vi "Collect Blueprints.vi"(1 "Blueprints List":string="Blueprint 1: Each ore robot costs 4 ore. Each clay robot costs 2 ore. Each obsidian robot costs 3 ore and 14 clay. Each geode robot costs 2 ore and 7 obsidian.\nBlueprint 2: Each ore robot costs 2 ore. Each clay robot costs 3 ore. Each obsidian robot costs 3 ore and 8 clay. Each geode robot costs 3 ore and 12 obsidian.") -> (0 "Blueprints":T1 {"Robot Building Costs"."Geode"."Mineral" items=["Ore", "Clay", "Obsidian", "Geode", "Open Geode"]; "Robot Building Costs"."Obsidian"."Mineral" items=["Ore", "Clay", "Obsidian", "Geode", "Open Geode"]; "Robot Building Costs"."Clay"."Mineral" items=["Ore", "Clay", "Obsidian", "Geode", "Open Geode"]; "Robot Building Costs"."Ore"."Mineral" items=["Ore", "Clay", "Obsidian", "Geode", "Open Geode"]})   [LabVIEW 2020, in "AoC 2022.lvlib"]
uses:
  AoC 2022.lvlib
  Blueprints.ctl
  Robot Building Costs.ctl
  Cost.ctl
  Mineral.ctl
  Mineral_Enum.ctl
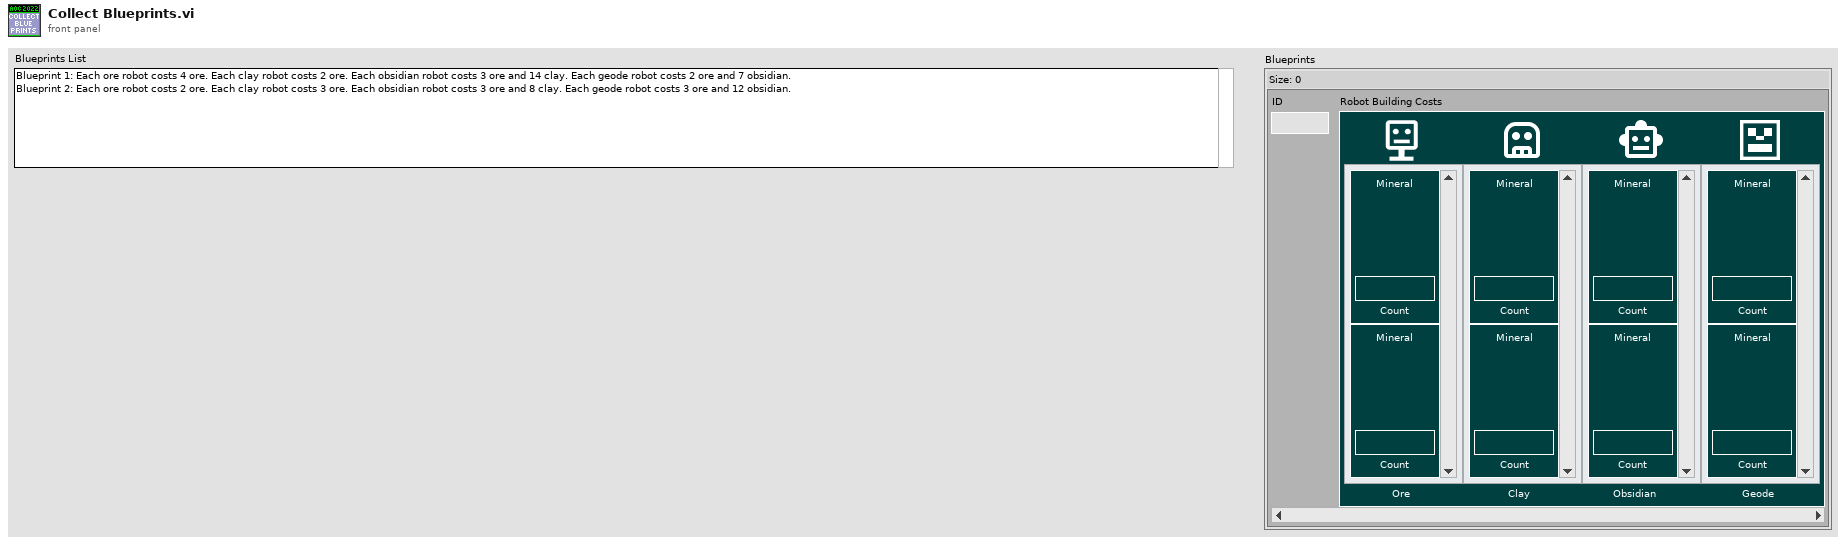
[diagram p1: front panel]
types:
  T1 = typedef "AoC 2022.lvlib/Blueprints.ctl" = map{i32, T2}
  T2 = typedef "AoC 2022.lvlib/Robot Building Costs.ctl" = cluster{"Ore":T3[], "Clay":T3[], "Obsidian":T3[], "Geode":T3[]}
  T3 = typedef "AoC 2022.lvlib/Cost.ctl" = cluster{"Mineral":T4, "Count":u32}
  T4 = typedef "AoC 2022.lvlib/Mineral.ctl" = u16
  T5 = typedef "AoC 2022.lvlib/Mineral_Enum.ctl" = enum16{"ore", "clay", "obsidian", "geode", "Open Geode"}
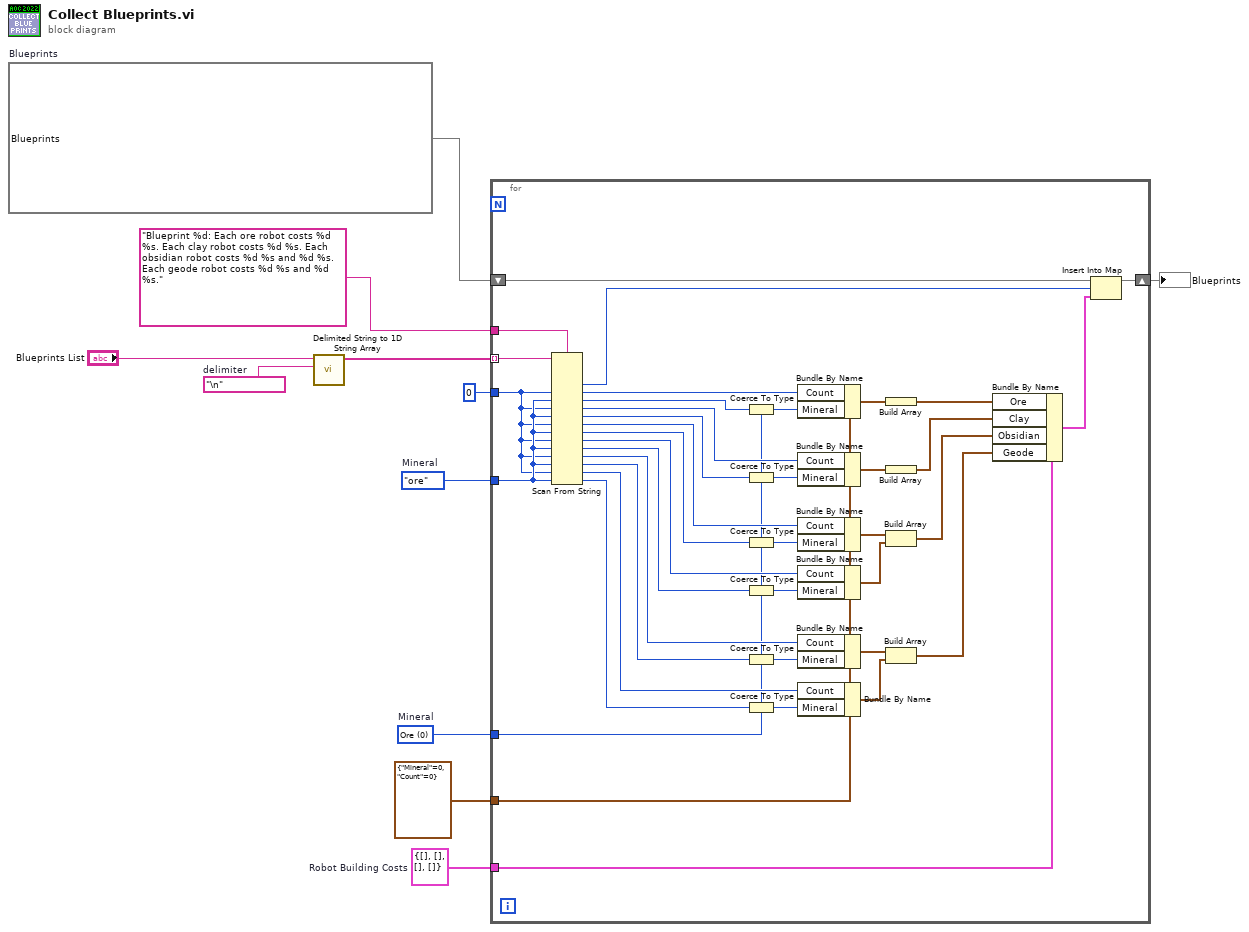
[diagram p0: block diagram]
diagram:
  w2 = T4 0 items=["Ore", "Clay", "Obsidian", "Geode", "Open Geode"]  # Mineral
  w4 = T2 {"Ore"=[], "Clay"=[], "Obsidian"=[], "Geode"=[]}  # Robot Building Costs
  w6 = T1 {}  # Blueprints
  w7 = Mineral_Enum."ore"  # Mineral
  w10 = "\n"  # delimiter
  n1 = call <vilib>:"Delimited String to 1D String Array.vi"("delimiter"=w10, "delimited string"="Blueprints List") -> ("string array"=w11:string[])  [unwired: 9 in]
  n2 = for {
    tunnel: w11 -> [w50] mode=indexing
    tunnel: "Blueprint %d: Each ore robot costs %d %s. Each clay robot costs %d %s. Each obsidian robot costs %d %s and %d %s. Each geode robot costs %d %s and %d %s." -> [w49]
    tunnel: w7 -> [w43]
    shift-right: [w47] -> w1
    shift-left: w6 -> [w48]
    tunnel: u32 0 -> [w22]
    tunnel: w4 -> [w45]
    tunnel: T3 {"Mineral"=0, "Count"=0} ("Cost") -> [w40]
    tunnel: w2 -> [w23]
    n3 = Scan From String(format string=w49, input string=w50, default 2=w22, default 3=w43, default 4=w22, default 5=w43, default 6=w22, default 7=w43, default 8=w22, default 9=w43, default 10=w22, default 11=w43, default 12=w22, default 13=w43) -> (output 1=w46:i32, output 2=w42:u32, output 3=w41:T5, output 4=w39:u32, output 5=w38:T5, output 6=w37:u32, output 7=w36:T5, output 8=w35:u32, output 9=w34:T5, output 10=w33:u32, output 11=w32:T5, output 12=w31:u32, output 13=w30:T5)  [unwired: 3 in, 3 out]
    n4 = Coerce To Type(0:w41, 1:w23) -> (2:w28:T4)
    n5 = Coerce To Type(0:w38, 1:w23) -> (2:w29:T4)
    n6 = Coerce To Type(0:w36, 1:w23) -> (2:w27:T4)
    n7 = Coerce To Type(0:w34, 1:w23) -> (2:w26:T4)
    n8 = Coerce To Type(0:w32, 1:w23) -> (2:w25:T4)
    n9 = Coerce To Type(0:w30, 1:w23) -> (2:w24:T4)
    n10 = Bundle By Name(cluster=w40, "Count"=w42, "Mineral"=w28) -> (w21:T3)
    n11 = Bundle By Name(cluster=w40, "Count"=w39, "Mineral"=w29) -> (w19:T3)
    n12 = Bundle By Name(cluster=w40, "Count"=w37, "Mineral"=w27) -> (w18:T3)
    n13 = Bundle By Name(cluster=w40, "Count"=w35, "Mineral"=w26) -> (w15:T3)
    n14 = Bundle By Name(cluster=w40, "Count"=w33, "Mineral"=w25) -> (w14:T3)
    n15 = Bundle By Name(cluster=w40, "Count"=w31, "Mineral"=w24) -> (w13:T3)
    n16 = Build Array(w21) -> (w20:T3[])
    n17 = Build Array(w19) -> (w17:T3[])
    n18 = Build Array(w18, w15) -> (w16:T3[])
    n19 = Build Array(w14, w13) -> (w12:T3[])
    n20 = Bundle By Name(cluster=w45, "Ore"=w20, "Clay"=w17, "Obsidian"=w16, "Geode"=w12) -> (w44:T2)
    n21 = Insert Into Map(map in=w48, key=w46, value=w44) -> (map out=w47:T1)  [unwired: 2 out]
  }
  "Blueprints" <- w1
